vi "ApplyLayoutToObject.vi"(5 "scaling settings":T1={"scaling factor"={"horizontal"=1.0, "vertical"=1.0}, "scale text"=FALSE} {"scaling factor"."vertical" min=0.0; "scaling factor"."horizontal" min=0.0}, 7 "properties to ignore":variant, 8 "error in (no error)":errorcluster, 10 "GObj Refnum":refnum<vi>, 11 "Text Decoration Layout in":refnum<class "Text Decoration Layout.lvclass">) -> (0 "error out":errorcluster, 3 "Text Decoration Layout out":refnum<class "Text Decoration Layout.lvclass">)   [LabVIEW 2010, in "NI_SE_Front Panel Layout.lvlib" / "Text Decoration Layout.lvclass"]
doc: "Apply layout information to the GObj Refnum."
uses:
  Text Decoration Layout.lvclass
  Scaling Factor_Options.ctl
  XY Scaling Factor.ctl
  Decoration Layout/Decoration Layout.lvclass
  Object Layout/Object Layout.lvclass/Object Layout.ctl
  Text Decoration Layout.lvclass/Text Decoration Layout.ctl
  Properties To Ignore.vi
  Set FP Object Size.vi
  NI_SE_Front Panel Layout.lvlib
  Object Layout/Object Layout.lvclass
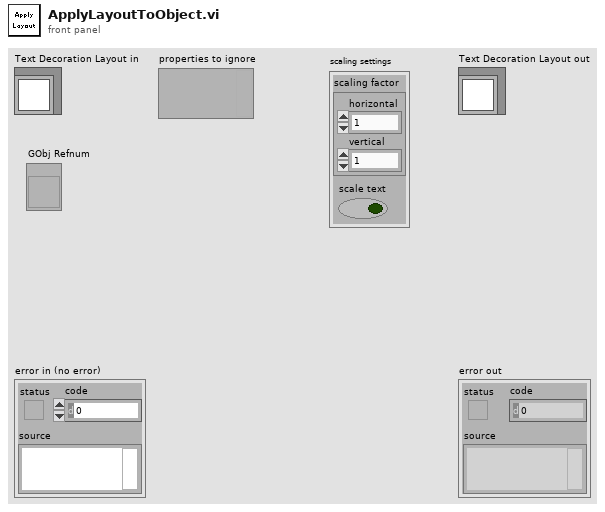
[diagram p1: front panel]
types:
  T1 = typedef "NI_SE_Front Panel Layout.lvlib/Scaling Factor_Options.ctl" = cluster{"scaling factor":T2, "scale text":bool}
  T2 = typedef "NI_SE_Front Panel Layout.lvlib/XY Scaling Factor.ctl" = cluster{"horizontal":dbl, "vertical":dbl}
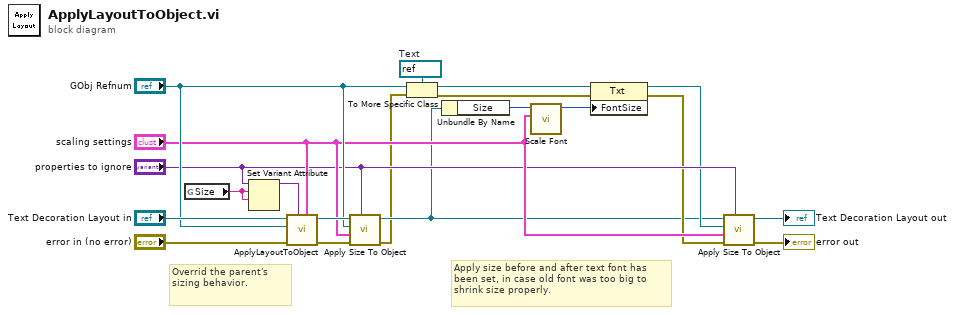
[diagram p0: block diagram]
diagram:
  w10 = refnum<vi> refnum  # Text
  # "Apply size before and after text font has been set, in case old font was too big to shrink size properly."
  # "Overrid the parent's sizing behavior."
  n1 = global read "Properties To Ignore.vi" "Size"() -> (w1:string)
  n2 = Set Variant Attribute(Variant="properties to ignore", name=w1, value=w1) -> (Variant out=w11:variant)  [unwired: 1 in, 2 out]
  n3 = call-parent "ApplyLayoutToObject.vi"("scaling settings"="scaling settings", "properties to ignore"=w11, "error in (no error)"="error in (no error)", "GObj Refnum"="GObj Refnum", "Decoration Layout in"="Text Decoration Layout in") -> ("error out"=w18:errorcluster, "Decoration Layout out"=w17:refnum<class "Text Decoration Layout.lvclass">)  [unwired: 5 in]
  n4 = call "Apply Size To Object.vi"("properties to ignore"="properties to ignore", "error in (no error)"=w18, "scaling settings"="scaling settings", "GObj Refnum"="GObj Refnum", "NI_SE_Object Layout in"=w17) -> ("error out"=w2:errorcluster, "NI_SE_Object Layout out"=w3:refnum<class "Text Decoration Layout.lvclass">)  [unwired: 5 in]
  n5 = To More Specific Class(target class=w10, reference="GObj Refnum", error in=w2) -> (specific class reference=w8:refnum<vi>, error out=w7:errorcluster)
  n6 = Unbundle By Name(w3) -> ("Size"=w9:u16)
  n7 = call "Scale Font.vi"("scaling settings"="scaling settings", "font size in"=w9) -> ("font size out"=w6:u16)  [unwired: 9 in]
  n8 = property class="Txt"(reference=w8, error in=w7, "FontSize"=w6) -> (reference out=w4:refnum<vi>, error out=w5:errorcluster)
  n9 = call "Apply Size To Object.vi"("properties to ignore"="properties to ignore", "error in (no error)"=w5, "scaling settings"="scaling settings", "GObj Refnum"=w4, "NI_SE_Object Layout in"=w3) -> ("error out"=→"error out":errorcluster, "NI_SE_Object Layout out"=→"Text Decoration Layout out":refnum<class "Text Decoration Layout.lvclass">)  [unwired: 5 in]
